vi "Main.vi"(8 "error out":errorcluster) -> (0 "error out 2":errorcluster)   [LabVIEW 2024]
doc: "This VI demonstrates how LabVIEW can use the drivers provided by MotioninJoy software to make full use of a Dualshock 3 Playstation 3 controller. It uses a type definition which allows a user to see direct button mapping."
uses:
  Controls/PS3 Controls.ctl
  backups BRIGHTLAB/CARNEVALI test3/Project_Brightlab_maschiatori/SLCMotors/FGV/FGV Actions.ctl
  <vilib>/Utility/inputDevices.llb/closeJoystick.vi
  <vilib>/ptbypt/NI_PtbyPt.lvlib
panel:
  in  "stop":bool
  out "PS3 Controls":T1 {"Left Analogue Stick X" scale=-32768.0..32768.0; "Left Analogue Stick Y" scale=32768.0..-32768.0; "Right Analogue Stick X" scale=-32768.0..32768.0; "Right Analogue Stick Y" scale=32768.0..-32768.0; "X Rotation" scale=-32768.0..32768.0; "Y Rotation" scale=-32768.0..32768.0; "L2 Pressure" scale=0.0..32768.0; "Numeric" format="%d°"}
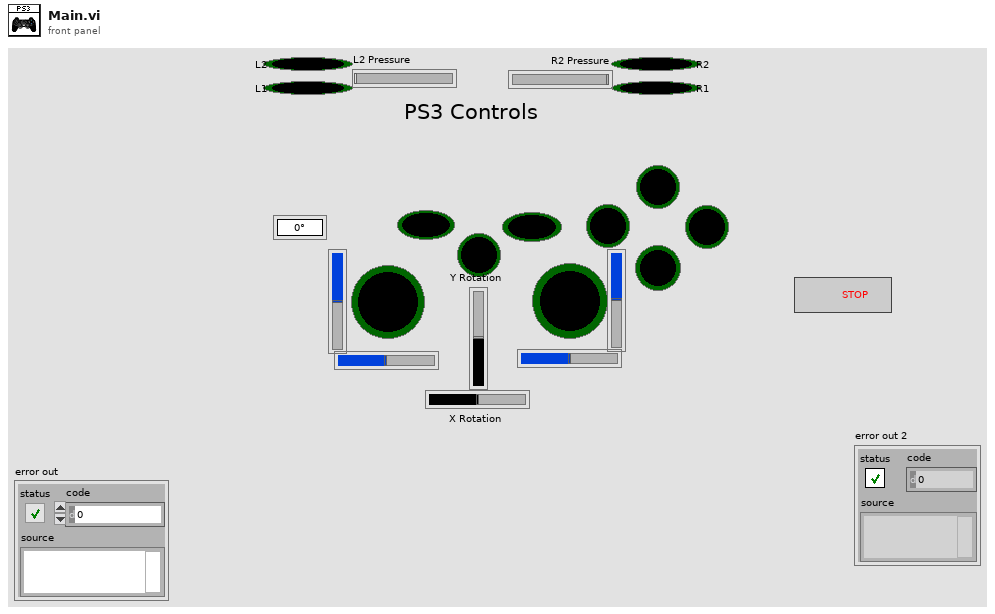
[diagram p1: front panel]
types:
  T1 = typedef "PS3 Controls.ctl" = cluster{"Left Analogue Stick X":i32, "Left Analogue Stick Y":i32, "Right Analogue Stick X":i32, "Right Analogue Stick Y":i32, "Y Rotation":i32, "X Rotation":i32, "L2 Pressure":i32, "R2 Pressure":i32, "Triangle":bool, "Circle":bool, "X":bool, "Square":bool, "L1":bool, "R1":bool, "L2":bool, "R2":bool, "L3":bool, "R3":bool, "Select":bool, "Start":bool, "PS Button":bool, "Numeric":i32}
  T2 = typedef "FGV Actions.ctl" = enum16{"Read", "Write"}
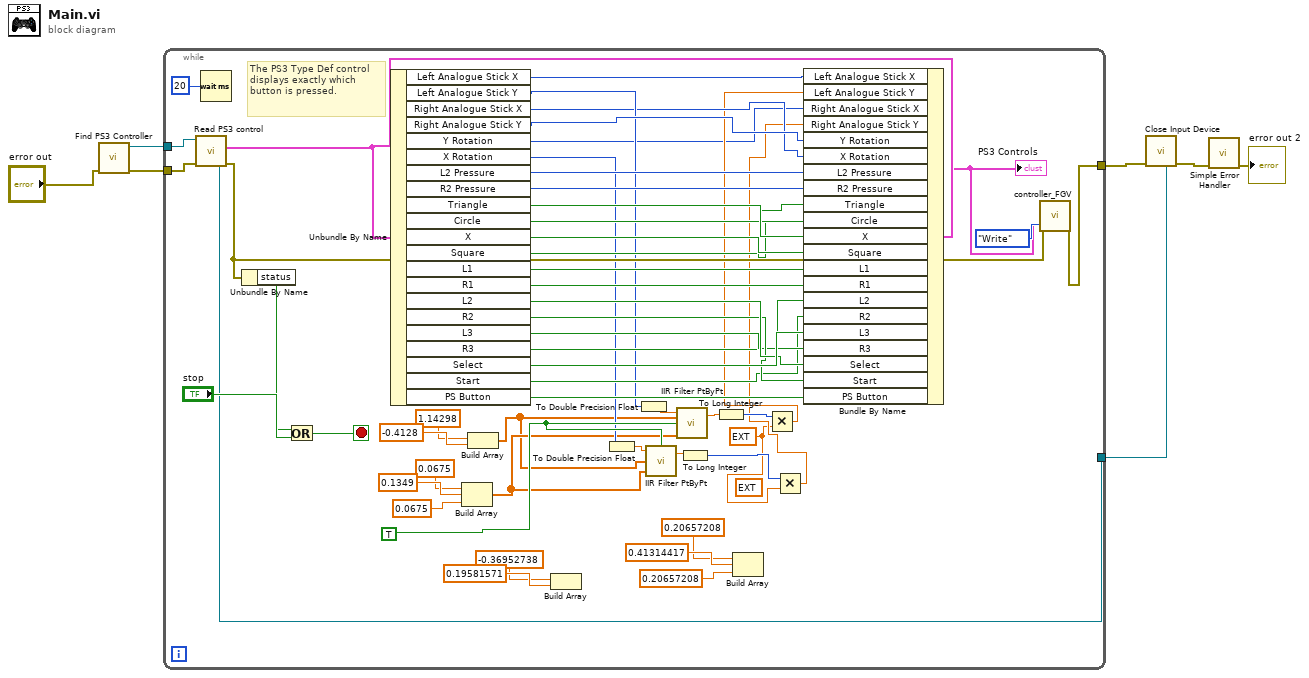
[diagram p0: block diagram]
diagram:
  n1 = call "Find PS3 Controller.vi"("error in (no error)"="error out") -> ("error out"=w7:errorcluster, "Controller Reference Out"=w6:refnum<k1>)  [unwired: 9 in]
  n2 = while {
    tunnel: w7 -> [w59]
    tunnel: w6 -> [w58]
    tunnel: [w57] -> w4
    tunnel: [w54] -> w1
    stop <- w61 stop-if-true
    (unwired) ext 1.78
    w8 = ext 15.9
    w23 = TRUE ("init/cont (init:F)")
    # "The PS3 Type Def control displays exactly which button is pressed."
    n3 = call "Read PS3 control.vi"("error in (no error)"=w59, "Controller Reference In"=w58) -> ("error out"=w55:errorcluster, "PS3 Controls"=w52:T1, "Controller Reference Out"=w57:refnum<k1>)  [unwired: 7 in]
    n4 = Wait (ms)(milliseconds to wait=u32 20) -> ()  [unwired: 1 out]
    n5 = Unbundle By Name(w55) -> ("status"=w56:bool)
    n6 = Or(x=w56, y="stop") -> (x .or. y?=w61:bool)
    n7 = Unbundle By Name(w52) -> ("Left Analogue Stick X"=w27:i32, "Left Analogue Stick Y"=w26:i32, "Right Analogue Stick X"=w22:i32, "Right Analogue Stick Y"=w28:i32, "Y Rotation"=w19:i32, "X Rotation"=w18:i32, "L2 Pressure"=w51:i32, "R2 Pressure"=w50:i32, "Triangle"=w45:bool, "Circle"=w44:bool, "X"=w43:bool, "Square"=w42:bool, "L1"=w41:bool, "R1"=w40:bool, "L2"=w48:bool, "R2"=w47:bool, "L3"=w46:bool, "R3"=w38:bool, "Select"=w49:bool, "Start"=w37:bool, "PS Button"=w39:bool)
    n8 = Build Array(0.0675 ("element"), 0.1349 ("element"), 0.0675 ("element")) -> (w10:dbl[])
    n9 = Build Array(1.14298 ("element"), -0.4128 ("element")) -> (w9:dbl[])
    n10 = Build Array(-0.36952738 ("element"), 0.19581571 ("element")) -> ()  [unwired: 1 out]
    n11 = To Double Precision Float(number=w18) -> (double precision float=w25:dbl)
    n12 = To Double Precision Float(number=w26) -> (double precision float=w30:dbl)
    n13 = call <vilib>:"IIR Filter PtByPt.vi"("initialize"=w23, "Forward Coefficients"=w10, "Reverse Coefficients"=w9, "x"=w25) -> ("Filtered x"=w24:dbl)  [unwired: 1 out]
    n14 = call <vilib>:"IIR Filter PtByPt.vi"("initialize"=w23, "Forward Coefficients"=w10, "Reverse Coefficients"=w9, "x"=w30) -> ("Filtered x"=w29:dbl)  [unwired: 1 out]
    n15 = To Long Integer(number=w24) -> (32bit integer=w12:i32)
    n16 = To Long Integer(number=w29) -> (32bit integer=w21:i32)
    n17 = Build Array(0.20657208 ("element"), 0.41314417 ("element"), 0.20657208 ("element")) -> ()  [unwired: 1 out]
    n18 = Multiply(x=w21, y=w8) -> (x*y=w20:ext)
    n19 = Multiply(x=w12, y=w8) -> (x*y=w11:ext)
    n20 = Bundle By Name(cluster=w52, "Left Analogue Stick X"=w27, "Left Analogue Stick Y"=w20, "Right Analogue Stick X"=w19, "Right Analogue Stick Y"=w11, "Y Rotation"=w28, "X Rotation"=w22, "L2 Pressure"=w51, "R2 Pressure"=w50, "Triangle"=w42, "Circle"=w44, "X"=w45, "Square"=w43, "L1"=w41, "R1"=w40, "L2"=w38, "R2"=w37, "L3"=w49, "R3"=w46, "Select"=w48, "Start"=w47, "PS Button"=w39) -> (w36:T1)
    "PS3 Controls" <- w36
    n21 = call "controller_FGV.vi"("error in"=w55, "PS3 Controls"=w36, "Action"=FGV_Actions."Write") -> ("error out"=w54:errorcluster)  [unwired: 8 in, 8 out]
  }
  n22 = call-poly <vilib>:"Close Input Device.vi"("error in (no error)"=w1, "device ID"=w4) -> ("error out"=w5:errorcluster)  [unwired: 8 in]
  n23 = call <vilib>:"Simple Error Handler.vi"("error in (no error)"=w5) -> ("error out"=→"error out 2":errorcluster)  [unwired: 4 in, 4 out]
